vi "Select window.vi"(0 "HP amount":T1(ring), 1 "Bullet amount":enum32{"2", "3", "4", "5", "6", "7", "8"}(ring), 2 "Item amount":enum32{"4", "5", "6"}(ring), 3 "Difficulty":u32(ring) items=["Easy", "Normal", "Hard"], 4 "Confirm":bool) -> ()   [LabVIEW 2025]
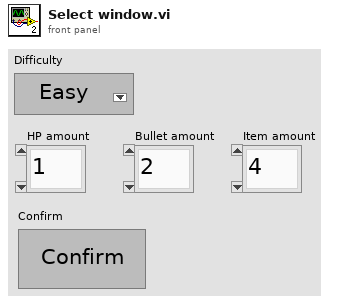
[diagram p1: front panel]
types:
  T1 = enum32{"1", "2", "3", "4", "5", "6", "7", "8", "9", "10"}
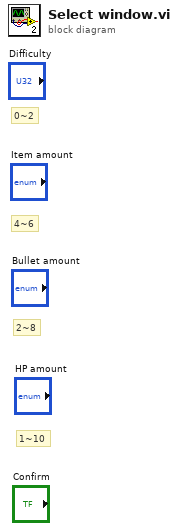
[diagram p0: block diagram]
diagram:
  # "1~10"
  # "0~2"
  # "2~8"
  # "4~6"
